vi "Unit Test.vi"() -> ()   [LabVIEW 2018]
uses:
  builds/Power_Supply.lvlibp/Power Supply.lvclass
panel:
  out "Output Out":bool
  out "Current Out":dbl
  out "Voltage Out":dbl
  in  "Output":bool
  in  "Current":dbl
  in  "Voltage":dbl
  out "error out":errorcluster
  in  "Stop":bool
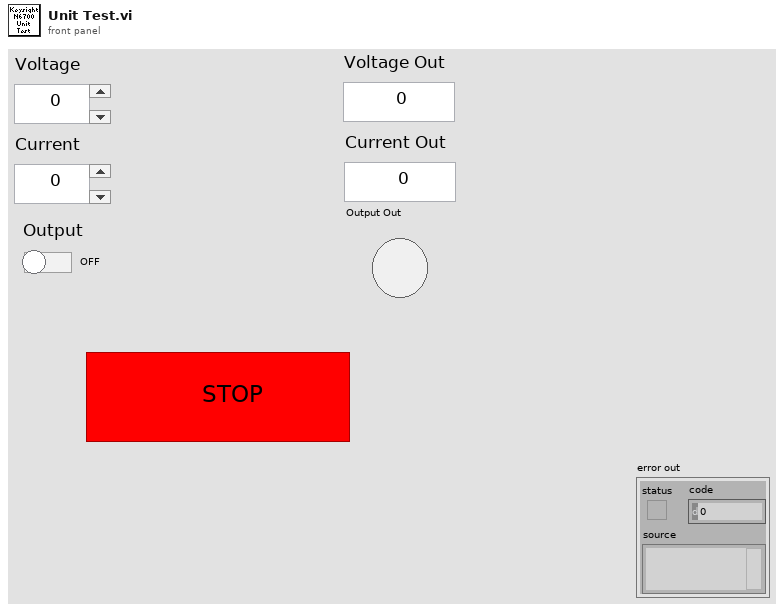
[diagram p1: front panel]
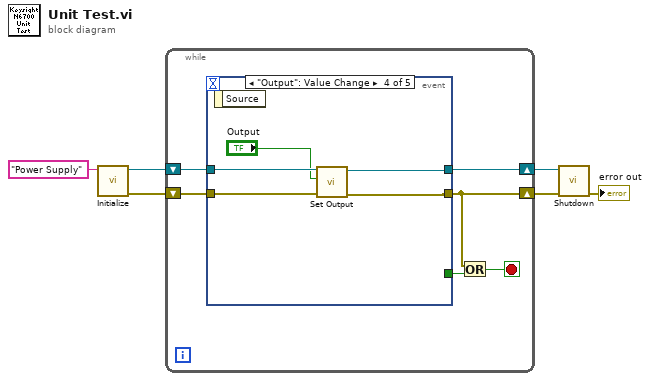
[diagram p0: block diagram]
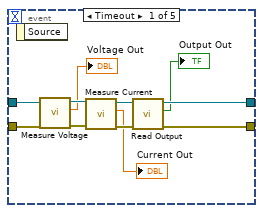
[diagram p2: hidden frame]
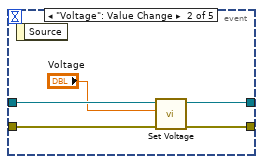
[diagram p3: hidden frame]
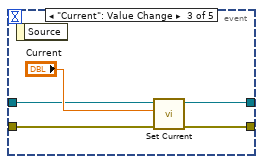
[diagram p4: hidden frame]
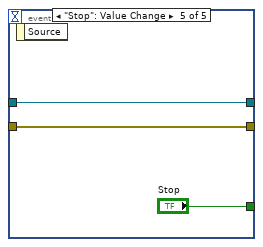
[diagram p5: hidden frame]
diagram:
  n1 = call "Initialize.vi"("Device"="Power Supply") -> ("error out"=w5:errorcluster, "Power Supply out"=w6:refnum<class "Power Supply.lvclass">)  [unwired: 9 in]
  n2 = while {
    shift-right: [w9] -> w4
    shift-left: w6 -> [w10]
    shift-right: [w7] -> w3
    shift-left: w5 -> [w8]
    stop <- w11 stop-if-true
    n3 = event shown="[3] \"Output\": Value Change" {
      selector: _ -> [_ _ _ _ _]
      dyn-events: _ -> [_ _ _ _ _]
      timeout: _ -> [_ _ _ _ _]
      tunnel: [_ _ _ _ "Stop"] -> w12
      tunnel: w10 -> [w16 w25 w29 w37 w40]
      tunnel: [w19 w26 w31 w36 w40] -> w9
      tunnel: w8 -> [w22 w28 w33 w38 w39]
      tunnel: [w20 w27 w32 w35 w39] -> w7
      event Timeout {
        n4 = event-data() -> ()  [unwired: 1 in, 1 out]
        n5 = call-dynamic "Measure Voltage.vi"("error in (no error)"=w22, "Power Supply in"=w16) -> ("error out"=w23:errorcluster, "Voltage"=→"Voltage Out":dbl, "Power Supply out"=w17:refnum<class "Power Supply.lvclass">)  [unwired: 7 in]
        n6 = call-dynamic "Measure Current.vi"("error in (no error)"=w23, "Power Supply in"=w17) -> ("error out"=w21:errorcluster, "Current"=→"Current Out":dbl, "Power Supply out"=w18:refnum<class "Power Supply.lvclass">)  [unwired: 7 in]
        n7 = call-dynamic "Read Output.vi"("error in"=w21, "Power Supply in"=w18) -> ("error out"=w20:errorcluster, "Output"=→"Output Out":bool, "Power Supply out"=w19:refnum<class "Power Supply.lvclass">)  [unwired: 7 in]
      }
      event "Voltage": Value Change {
        n8 = event-data() -> ()  [unwired: 1 in, 1 out]
        n9 = call "Set Voltage.vi"("error in"=w28, "Voltage"="Voltage", "Power Supply in"=w25) -> ("error out"=w27:errorcluster, "Power Supply out"=w26:refnum<class "Power Supply.lvclass">)  [unwired: 7 in]
      }
      event "Current": Value Change {
        n10 = event-data() -> ()  [unwired: 1 in, 1 out]
        n11 = call "Set Current.vi"("error in"=w33, "Current"="Current", "Power Supply in"=w29) -> ("error out"=w32:errorcluster, "Power Supply out"=w31:refnum<class "Power Supply.lvclass">)  [unwired: 7 in]
      }
      event "Output": Value Change {
        n12 = event-data() -> ()  [unwired: 1 in, 1 out]
        n13 = call "Set Output.vi"("error in"=w38, "Output"="Output", "Power Supply in"=w37) -> ("error out"=w35:errorcluster, "Power Supply out"=w36:refnum<class "Power Supply.lvclass">)  [unwired: 7 in]
      }
      event "Stop": Value Change {
        n14 = event-data() -> ()  [unwired: 1 in, 1 out]
      }
    }
    n15 = Or(x=w7, y=w12) -> (x .or. y?=w11:bool)
  }
  n16 = call "Shutdown.vi"("error in"=w3, "Power Supply in"=w4) -> ("error out"=→"error out":errorcluster)  [unwired: 8 in, 1 out]
